vi "ui_ClientSrv Query Machine and Port.vi"() -> (4 "OKed?":bool, 6 "machine name out":string, 8 "port number out":u32)   [LabVIEW 2012]
doc: "This dialog allows entry of information required to connect to a server. The password is separately queried. Once a succesful connection is established, the client will add the server and its connection information to its list of server presets or update any matching outdated preset."
uses:
  typedefs/t_ClientSrv Query Machine and Port States.ctl
panel:
  in  "port number":u32=3363
  in  "machine name or IP address":string
  in  "cancel":bool
  in  "OK":bool
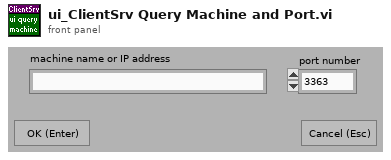
[diagram p1: front panel]
types:
  T1 = typedef "t_ClientSrv Query Machine and Port States.ctl" = enum16{"empty queue", "initialize", "stop"}
  T2 = typedef "eventvkey.ctl" = enum16{"ASCII", "Enter", "Return", "Shift", "Ctrl", "Alt", "Cmd", "Opt", "Caps", "NumLock", "Clear", "Break", "Up", "Down", "Left", "Right", "Insert", "Delete", "Home", "End", "PageUp", "PageDown", "Escape", "Help", "Pause", "ScrollLock", "F1", "F2", "F3", "F4", "F5", "F6", "F7", "F8", "F9", "F10", "F11", "F12", "F13", "F14", "F15", "F16", "F17", "F18", "F19", "F20", "F21", "F22", "F23", "F24", "Play", "VolumeUp", "VolumeDown", "Mute", "Two Byte Char"}
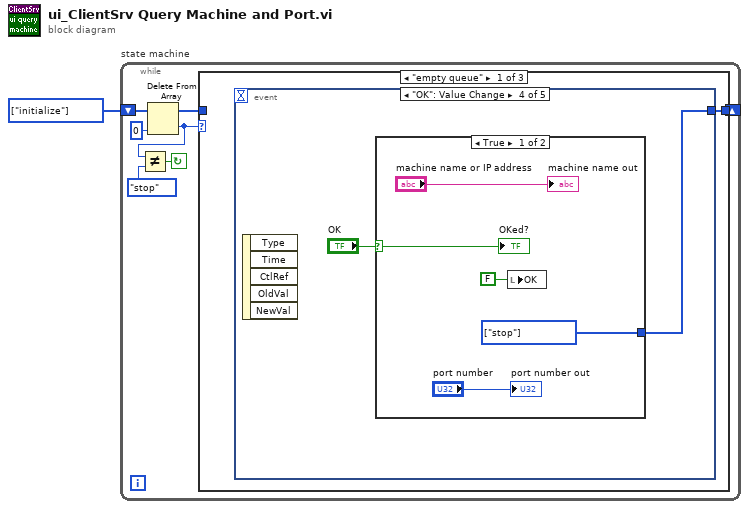
[diagram p0: block diagram]
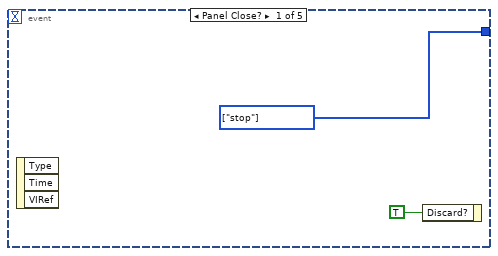
[diagram p2: hidden frame]
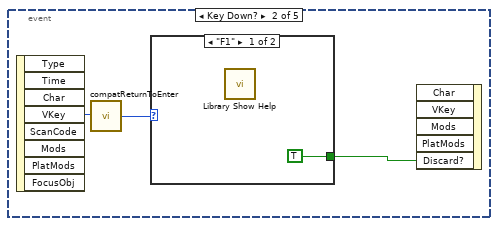
[diagram p3: hidden frame]
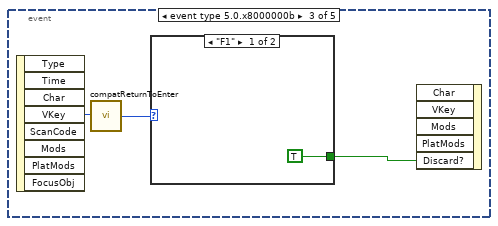
[diagram p5: hidden frame]
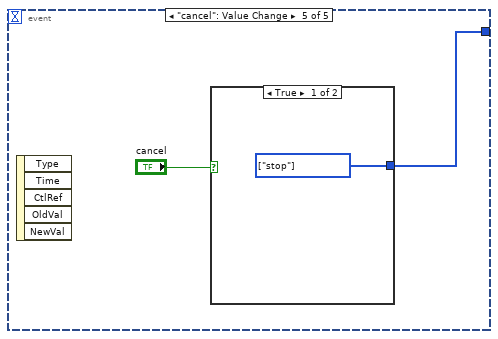
[diagram p8: hidden frame]
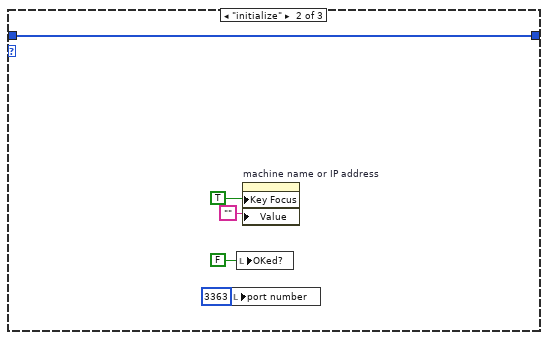
[diagram p10: hidden frame]
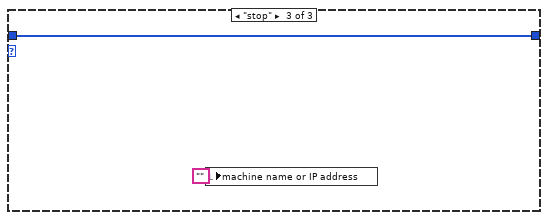
[diagram p11: hidden frame]
diagram:
  w1 = T1[] [enum."initialize"] items=["empty queue", "initialize", "stop"] ("Array Constant")
  n1 = while "state machine" {
    shift-left: w1 -> [w5]
    shift-right: [w8] -> _
    stop <- w7 continue-if-true
    n2 = Delete From Array(array=w5, index=0) -> (deleted portion=w3:T1, array with subset deleted=w4:T1[])  [unwired: 1 in]
    n3 = Not Equal?(x=w3, y=t_ClientSrv_Query_Machine_and_Port_States."stop" ("states")) -> (x != y?=w7:bool)
    n4 = case "Case" shown="\"empty queue\"" w3 {
      tunnel: [w9 w34 w36] -> w8
      tunnel: w4 -> [_ w34 w36]
      frame "empty queue" {
        n5 = event shown="[3] \"OK\": Value Change" {
          selector: _ -> [_ _ _ _ _]
          dyn-events: _ -> [_ _ _ _ _]
          timeout: _ -> [_ _ _ _ _]
          tunnel: [w11 _ _ w21 w28] -> w9
          event Panel Close? {
            w11 = T1[] [enum."stop"] items=["empty queue", "initialize", "stop"] ("Array Constant")
            n6 = event-data() -> ()  [unwired: 1 in, 3 out]
            n7 = event-data("Discard?"=TRUE) -> ()  [unwired: 1 in, 1 out]
          }
          event Key Down? {
            n8 = event-data() -> ("VKey"=w12:T2)  [unwired: 1 in, 7 out]
            n9 = call <vilib>:"compatReturnToEnter.vi"("VKey"=w12) -> ("VKey"=w14:T2)
            n10 = case shown="\"F1\"" w14 {
              tunnel: [TRUE ("Discard?") _] -> w13
              frame "F1" {
                n11 = call "Library Show Help.vi"() -> ()  [unwired: 1 in]
              }
              frame Default {
              }
            }
            n12 = event-data("Discard?"=w13) -> ()  [unwired: 5 in, 1 out]
          }
          event event type 5.0.x8000000b {
            n13 = event-data() -> ("VKey"=w16:T2)  [unwired: 1 in, 7 out]
            n14 = call <vilib>:"compatReturnToEnter.vi"("VKey"=w16) -> ("VKey"=w18:T2)
            n15 = case shown="\"F1\"" w18 {
              tunnel: [TRUE ("Discard?") _] -> w17
              frame "F1" {
              }
              frame Default {
              }
            }
            n16 = event-data("Discard?"=w17) -> ()  [unwired: 5 in, 1 out]
          }
          event "OK": Value Change {
            n17 = event-data() -> ()  [unwired: 1 in, 5 out]
            n18 = case shown="True" "OK" {
              selector: "OK" -> [w25 _]
              tunnel: [w26 _] -> w21
              frame True {
                w26 = T1[] [enum."stop"] items=["empty queue", "initialize", "stop"] ("Array Constant")
                n19 = local write "OK"(FALSE ("OK")) -> ()
                "OKed?" <- w25
                "machine name out" <- "machine name or IP address"
                "port number out" <- "port number"
              }
              frame False {
              }
            }
          }
          event "cancel": Value Change {
            n20 = event-data() -> ()  [unwired: 1 in, 5 out]
            n21 = case shown="True" "cancel" {
              tunnel: [w29 _] -> w28
              frame True {
                w29 = T1[] [enum."stop"] items=["empty queue", "initialize", "stop"] ("Array Constant")
              }
              frame False {
              }
            }
          }
        }
      }
      frame "initialize" {
        n22 = local write "port number"(u32 3363 ("port number")) -> ()
        n23 = local write "OKed?"(FALSE ("OKed?")) -> ()
        n24 = property on="machine name or IP address" class="Str"("Key Focus"=TRUE, "Value"="" ("machine name")) -> ()  [unwired: 2 in, 2 out]
      }
      frame "stop" {
        n25 = local write "machine name or IP address"("" ("machine name or IP address")) -> ()
      }
    }
  }
